vi "Create Directory Chain.vi"(8 "Error In":errorcluster, 11 "Path":path) -> (0 "Error Out":errorcluster, 3 "Duplicate Path":path)   [LabVIEW 2020]
doc: "Create a directory and its parent directories if necessary.\n\nFreeware from Moore Good Ideas, www.mooregoodideas.com. Do not remove this line."
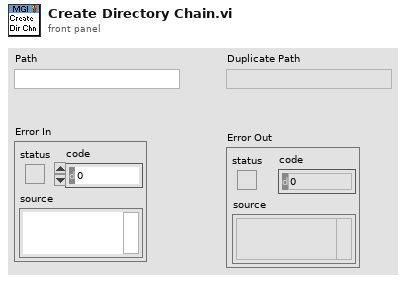
[diagram p1: front panel]
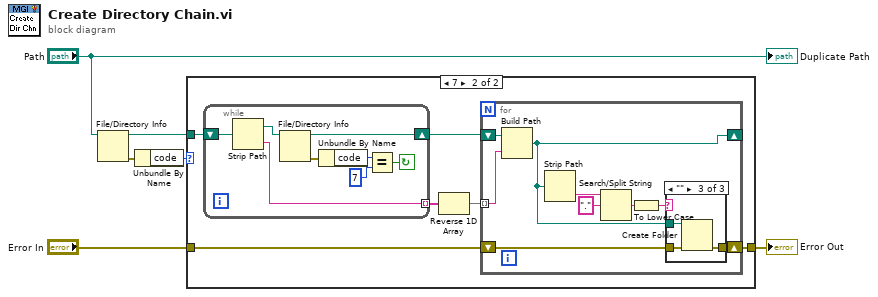
[diagram p0: block diagram]
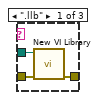
[diagram p3: hidden frame]
diagram:
  n1 = File/Directory Info(path="Path") -> (path out=w1:path, error out=w4:errorcluster)  [unwired: 1 in, 5 out]
  n2 = Unbundle By Name(w4) -> ("code"=w3:i32)
  n3 = case shown="7" w3 {
    tunnel: "Error In" -> [w7 w10]
    tunnel: [w7 w9] -> w6
    tunnel: w1 -> [_ w8]
    frame Default {
    }
    frame 7 {
      n4 = while {
        shift-right: [w30] -> w12
        shift-left: w8 -> [w37]
        tunnel: [w31] -> w13 mode=indexing
        stop <- w32 continue-if-true
        n5 = Strip Path(path=w37) -> (stripped path=w36:path, name=w31:string)
        n6 = File/Directory Info(path=w36) -> (path out=w30:path, error out=w35:errorcluster)  [unwired: 1 in, 5 out]
        n7 = Unbundle By Name(w35) -> ("code"=w34:i32)
        n8 = Equal?(x=w34, y=7) -> (x = y?=w32:bool)
      }
      n9 = Reverse 1D Array(array=w13) -> (reversed array=w11:string[])
      n10 = for {
        shift-right: [w14] -> _
        shift-left: w12 -> [w22]
        tunnel: w11 -> [w21] mode=indexing
        shift-right: [w19] -> w9
        shift-left: w10 -> [w20]
        n11 = Build Path(base path=w22, name or relative path=w21) -> (appended path=w14:path)
        n12 = Strip Path(path=w14) -> (name=w16:string)  [unwired: 1 out]
        n13 = Search/Split String(string=w16, search string/char (-)="." ("search char (-)")) -> (match + rest of string=w17:string)  [unwired: 1 in, 2 out]
        n14 = To Lower Case(string=w17) -> (all lower case string=w15:string)
        n15 = case shown="\"\"" w15 {
          tunnel: w20 -> [w25 w26 w29]
          tunnel: w14 -> [w24 _ w28]
          tunnel: [w23 w26 w27] -> w19
          frame ".llb" {
            n16 = call <vilib>:"New VI Library.vi"("error in (no error)"=w25, "VI library path in"=w24) -> ("error out"=w23:errorcluster)  [unwired: 8 in, 1 out]
          }
          frame Default {
          }
          frame "" {
            n17 = Create Folder(path (use dialog)=w28, error in=w29) -> (error out=w27:errorcluster)  [unwired: 1 in, 2 out]
          }
        }
      }
    }
  }
  "Error Out" <- w6
  "Duplicate Path" <- "Path"
